vi "RPM_From_Lookup.vi"() -> (0 "RPM output":dbl, 1 "Array Index":dbl, 2 "Fractional Index":dbl, 3 "Search Value":dbl)   [LabVIEW 2019]
uses:
  Globals/Flywheel_Globals.vi
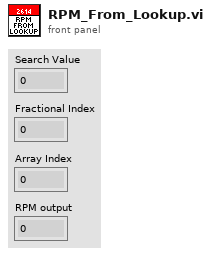
[diagram p1: front panel]
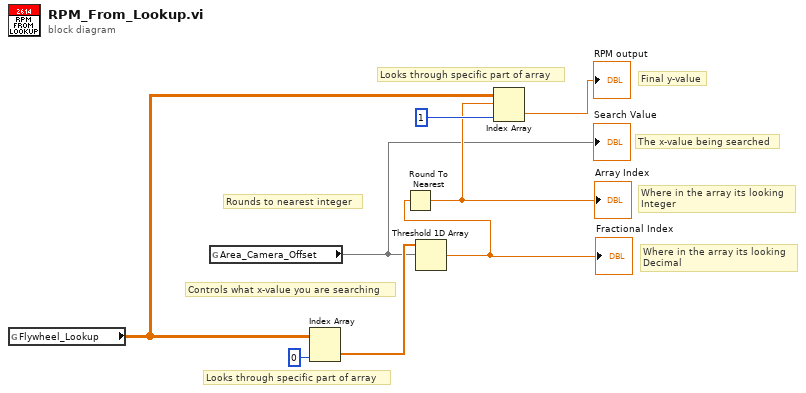
[diagram p0: block diagram]
diagram:
  # "Looks through specific part of array"
  # "Looks through specific part of array"
  # "Rounds to nearest integer"
  # "Controls what x-value you are searching"
  # "The x-value being searched"
  # "Where in the array its looking\nInteger"
  # "Where in the array its looking\nDecimal"
  # "Final y-value"
  n1 = global read "Flywheel_Globals.vi" "Flywheel_Lookup"() -> (w2:dbl[][])
  n2 = global read "Flywheel_Globals.vi" "Area_Camera_Offset"() -> (w1)
  "Search Value" <- w1
  n3 = Index Array(array=w2, index (col)=0 ("disabled index (col)")) -> (element=w7:dbl[])  [unwired: 1 in]
  n4 = Threshold 1D Array(2:w1, 3:w7) -> (0:w6:dbl)  [unwired: 1 in]
  "Fractional Index" <- w6
  n5 = Round To Nearest(number=w6) -> (nearest integer value=w3:dbl)
  "Array Index" <- w3
  n6 = Index Array(array=w2, index (row)=w3, index (col)=1 ("disabled index (row)")) -> (element=→"RPM output":dbl)
